vi "Read Sensor (sub VI).vi"(0 "Input cluster":T1) -> (1 "Reading":dbl, 2 "Output cluster":T1)   [LabVIEW 2016]
doc: "Send the Read command (R/r) to an Atlas sensor, wait for 800ms and read the response"
uses:
  Visa com cluster def (subVI).ctl
panel:
  out "read buffer":string
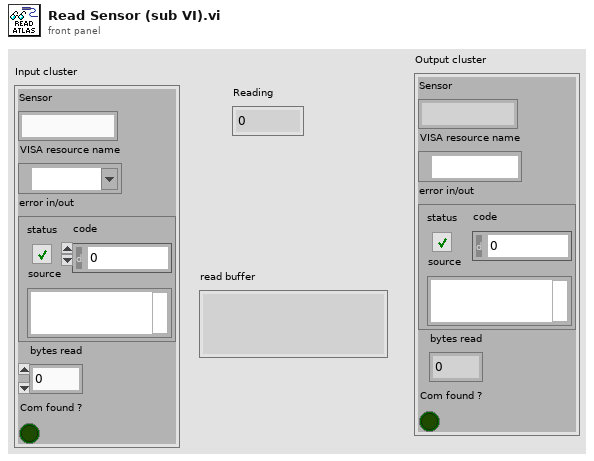
[diagram p1: front panel]
types:
  T1 = typedef "Visa com cluster def (subVI).ctl" = cluster{"Sensor":string, "VISA resource name":refnum<visa-resource-name>, "error in/out":errorcluster, "bytes read":u32, "Com found ?":bool}
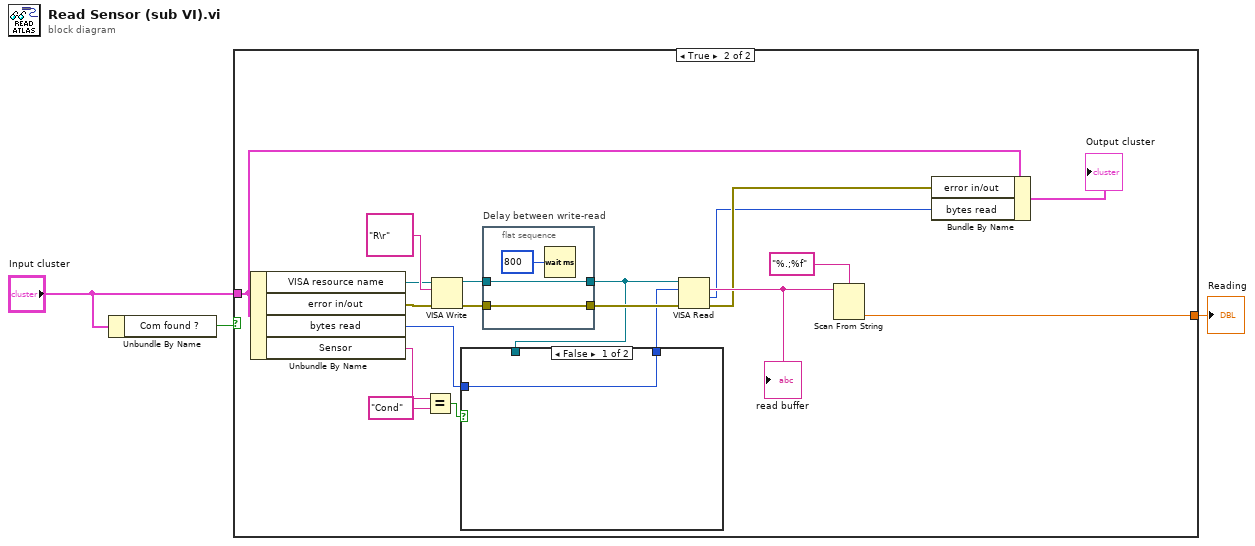
[diagram p0: block diagram]
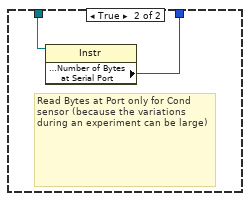
[diagram p3: hidden frame]
diagram:
  n1 = Unbundle By Name("Input cluster") -> ("Com found ?"=w3:bool)
  n2 = case shown="True" w3 {
    tunnel: "Input cluster" -> [_ w14]
    tunnel: [_ w16] -> w1
    frame False {
    }
    frame True {
      n3 = Unbundle By Name(w14) -> ("VISA resource name"=w8:refnum<visa-resource-name>, "error in/out"=w17:errorcluster, "bytes read"=w9:u32, "Sensor"=w11:string)
      n4 = Equal?(x=w11, y="Cond") -> (x = y?=w12:bool)
      n5 = VISA Write(VISA resource name=w8, write buffer="R\r" ("Command (RT\\r, RS\\r)"), error in (no error)=w17) -> (VISA resource name out=w6:refnum<visa-resource-name>, error out=w18:errorcluster)  [unwired: 1 out]
      n6 = case shown="False" w12 {
        tunnel: w9 -> [w23 _]
        tunnel: w5 -> [_ w25]
        tunnel: [w23 w24] -> w7
        frame False {
        }
        frame True {
          # "Read Bytes at Port only for Cond sensor (because the variations during an experiment can be large)"
          n7 = property class="Instr"(reference=w25) -> ("Serial Settings:Number of Bytes at Serial Port"=w24:u32)  [unwired: 1 in, 2 out]
        }
      }
      n8 = flat-sequence "Delay between write-read" {
        tunnel: w18 -> [w28]
        tunnel: [w28] -> w19
        tunnel: w6 -> [w27]
        tunnel: [w27] -> w5
        frame #0 {
          n9 = Wait (ms)(milliseconds to wait=u32 800 ("delay before read (ms)")) -> ()  [unwired: 1 out]
        }
      }
      n10 = VISA Read(VISA resource name=w5, byte count=w7, error in (no error)=w19) -> (read buffer=w21:string, return count=w4:u32, error out=w13:errorcluster)  [unwired: 1 out]
      "read buffer" <- w21
      n11 = Scan From String(format string="%.;%f" ("format"), input string=w21) -> (output 1=w16:dbl)  [unwired: 3 in, 3 out]
      n12 = Bundle By Name(cluster=w14, "error in/out"=w13, "bytes read"=w4) -> (→"Output cluster":T1)
    }
  }
  "Reading" <- w1
